vi "Test Read Booleans.vi"(11 "TwinCAT ADS in":refnum<class "TwinCAT ADS.lvclass">) -> (3 "TwinCAT ADS out":refnum<class "TwinCAT ADS.lvclass">)   [LabVIEW 2018]
uses:
  TwinCAT ADS Class/TwinCAT ADS.lvclass
  0e82c4fa-873b-4361-ac99-2e6e4b7cd392.vi
  da0f88be-82f8-4e5b-86e7-5baa69d9b51e.vi
  4782b519-43e7-4b8e-bd72-e209be860882.vi
  e7a7b24b-aede-49d7-b369-bb451e1de87e.vi
  TwinCAT ADS Class/VIs/Data/Read.vi
  <vilib>/addons/_JKI Toolkits/Caraya/classes/Assert/Assert True.vi
  <vilib>/addons/_JKI Toolkits/Caraya/classes/Assert/Assert.lvclass
  <vilib>/addons/_JKI Toolkits/Caraya/classes/Test/Test.lvclass
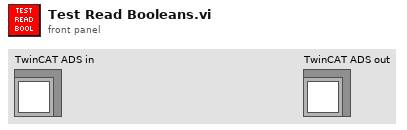
[diagram p1: front panel]
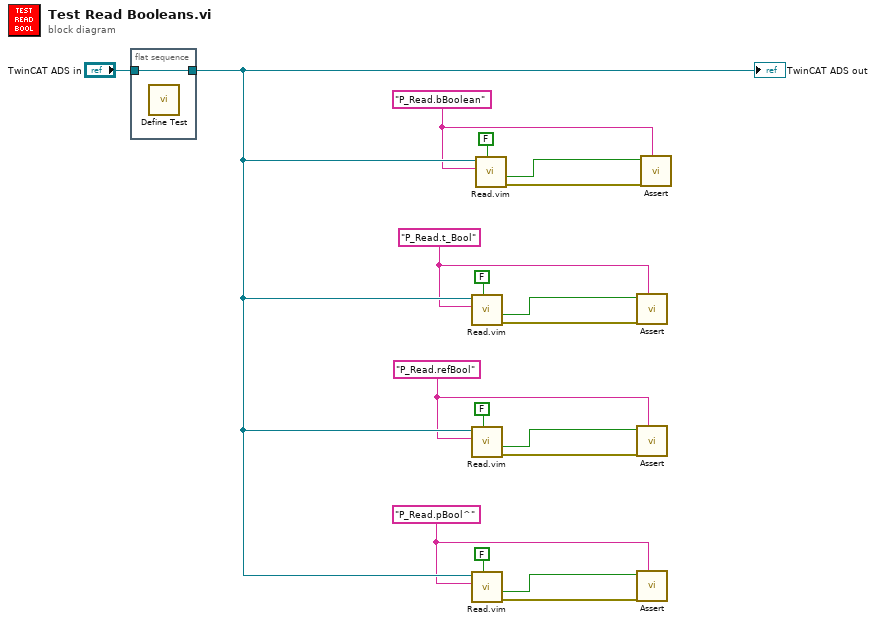
[diagram p0: block diagram]
diagram:
  w4 = "P_Read.pBool^" ("Symbol Name")
  w5 = "P_Read.refBool" ("Symbol Name")
  w12 = "P_Read.t_Bool" ("Symbol Name")
  w13 = "P_Read.bBoolean" ("Symbol Name")
  n1 = flat-sequence {
    tunnel: "TwinCAT ADS in" -> [w19]
    tunnel: [w19] -> w18
    frame #0 {
      n2 = call <vilib>:"Define Test.vi"() -> ()  [unwired: 10 in, 2 out]
    }
  }
  n3 = call "Read.vim"("Type"=FALSE, "Symbol Name"=w12, "TwinCAT ADS in"=w18) -> ("error out"=w10:errorcluster, "Value"=w11:bool)  [unwired: 6 in, 1 out]
  n4 = call "Read.vim"("Type"=FALSE, "Symbol Name"=w5, "TwinCAT ADS in"=w18) -> ("error out"=w7:errorcluster, "Value"=w6:bool)  [unwired: 6 in, 1 out]
  n5 = call "Read.vim"("Type"=FALSE, "Symbol Name"=w4, "TwinCAT ADS in"=w18) -> ("error out"=w2:errorcluster, "Value"=w3:bool)  [unwired: 6 in, 1 out]
  n6 = call "Read.vim"("Type"=FALSE, "Symbol Name"=w13, "TwinCAT ADS in"=w18) -> ("error out"=w16:errorcluster, "Value"=w15:bool)  [unwired: 6 in, 1 out]
  n7 = call-poly <vilib>:"Assert.vi"("Label"=w12, "error in (no error)"=w10, "True?"=w11) -> ()  [unwired: 7 in, 2 out]
  n8 = call-poly <vilib>:"Assert.vi"("Label"=w5, "error in (no error)"=w7, "True?"=w6) -> ()  [unwired: 7 in, 2 out]
  n9 = call-poly <vilib>:"Assert.vi"("Label"=w4, "error in (no error)"=w2, "True?"=w3) -> ()  [unwired: 7 in, 2 out]
  n10 = call-poly <vilib>:"Assert.vi"("Label"=w13, "error in (no error)"=w16, "True?"=w15) -> ()  [unwired: 7 in, 2 out]
  "TwinCAT ADS out" <- w18
